vi "Convert CAN Frame.vi"(8 "error in (no error)":errorcluster, 9 "timestamp":timestamp, 10 "CAN frame":T1 {"type" items=["CAN Data", "CAN Remote"]; "identifier" format="%.0x"}, 11 "tdms file":refnum<k34>) -> (0 "error out":errorcluster, 3 "tdms file out":refnum<k34>)   [LabVIEW 2014]
uses:
  <vilib>/RioEmbeddedCAN/RioEmbeddedCAN.llb/CANFrameControl.ctl
  TDMS Timestamp and Data Double.vi
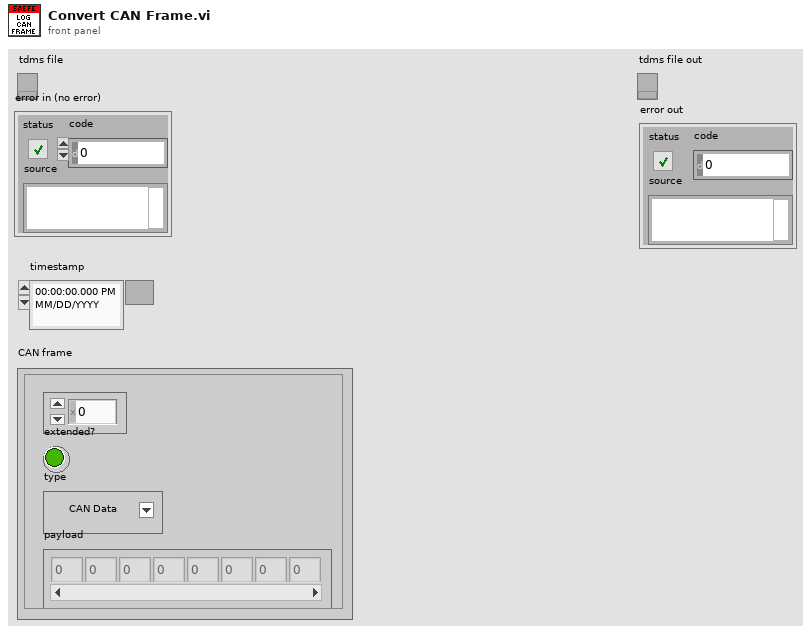
[diagram p1: front panel]
types:
  T1 = typedef "CANFrameControl.ctl" = cluster{"identifier":u32, "extended?":bool, "type":u8, "payload":u8[]}
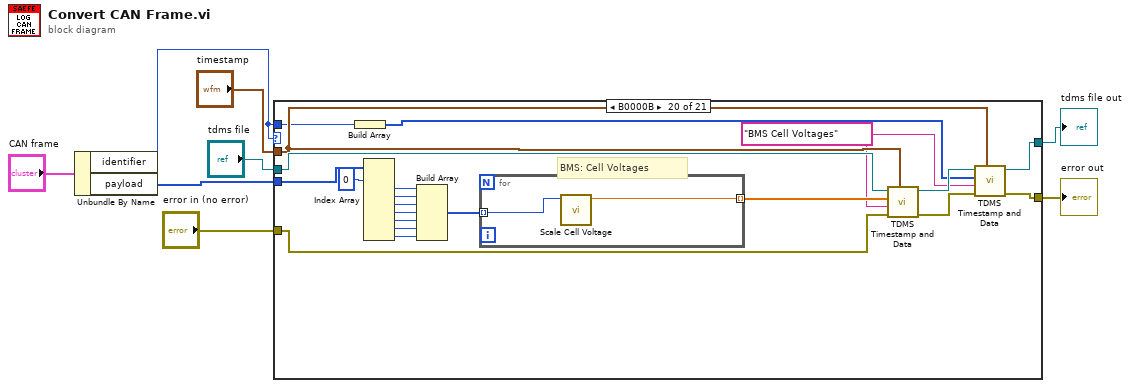
[diagram p0: block diagram]
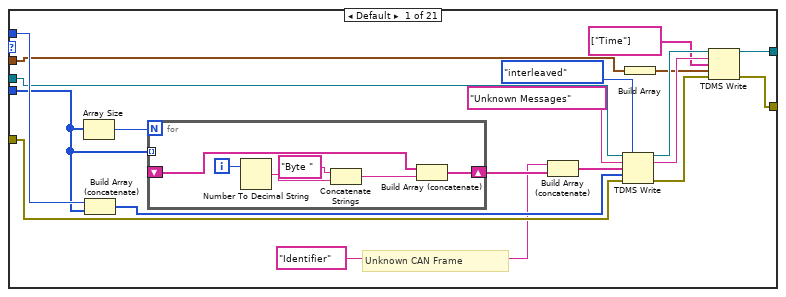
[diagram p2: hidden frame]
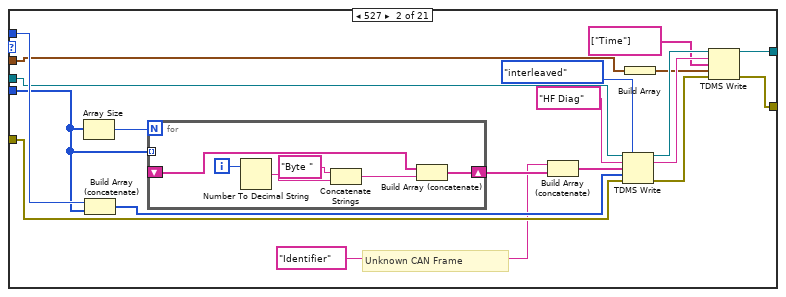
[diagram p3: hidden frame]
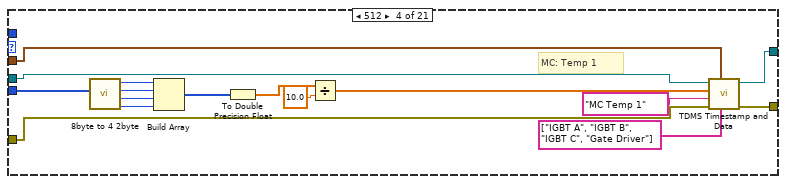
[diagram p5: hidden frame]
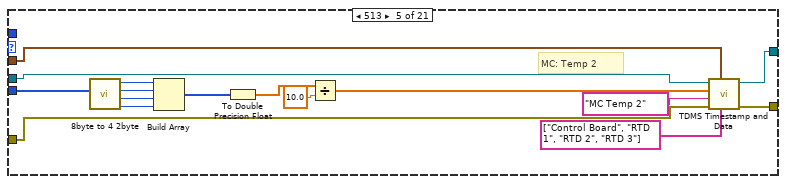
[diagram p6: hidden frame]
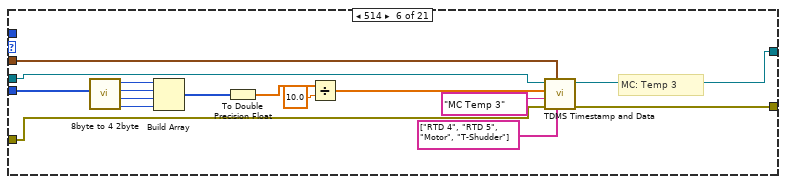
[diagram p7: hidden frame]
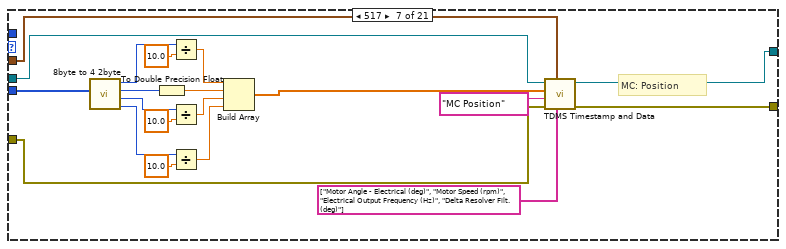
[diagram p8: hidden frame]
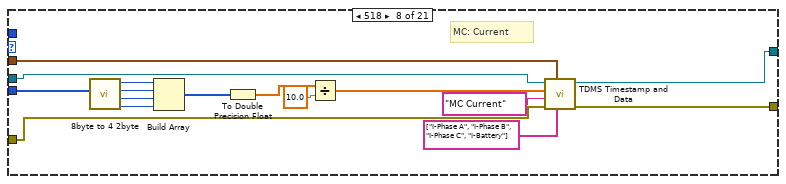
[diagram p9: hidden frame]
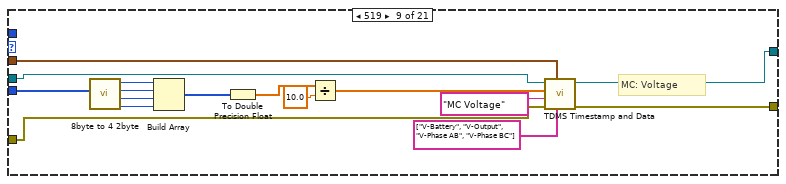
[diagram p10: hidden frame]
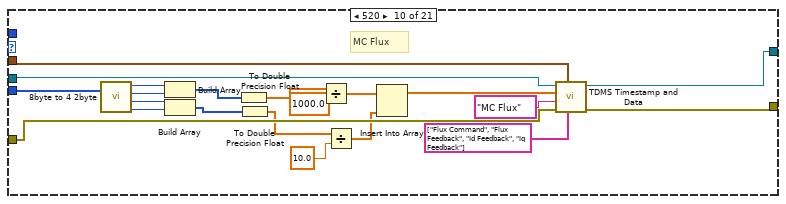
[diagram p11: hidden frame]
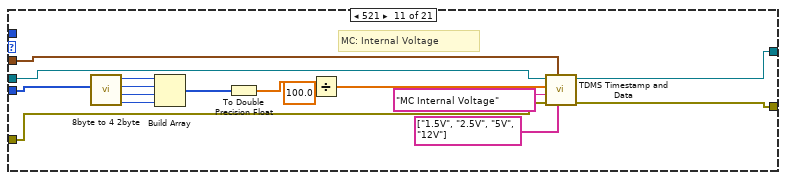
[diagram p12: hidden frame]
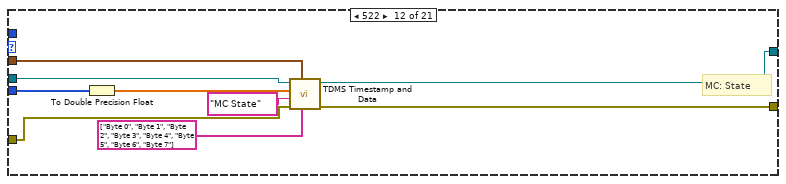
[diagram p13: hidden frame]
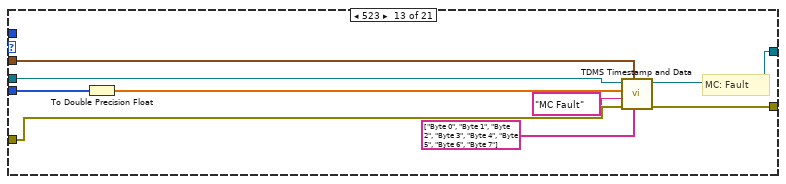
[diagram p14: hidden frame]
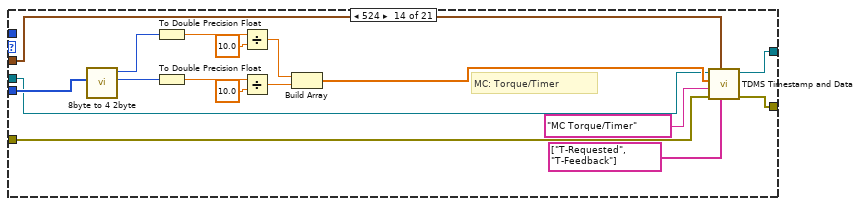
[diagram p15: hidden frame]
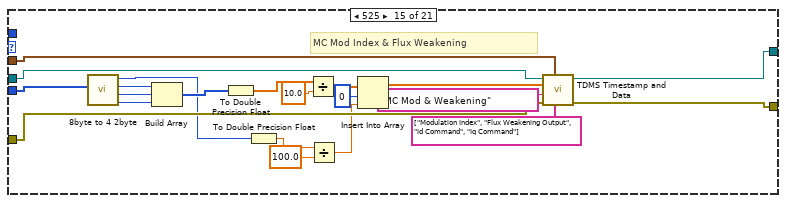
[diagram p16: hidden frame]
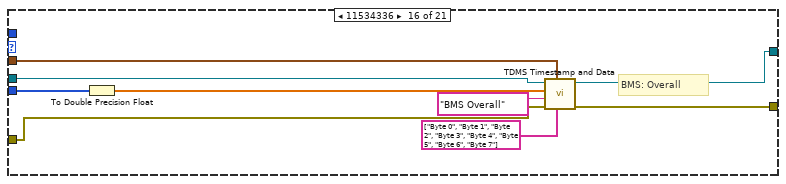
[diagram p17: hidden frame]
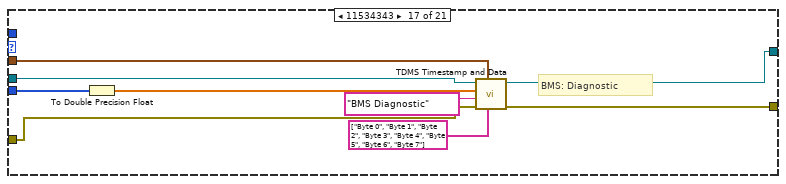
[diagram p18: hidden frame]
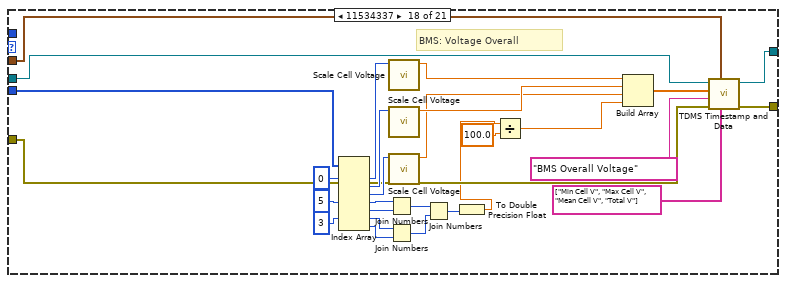
[diagram p19: hidden frame]
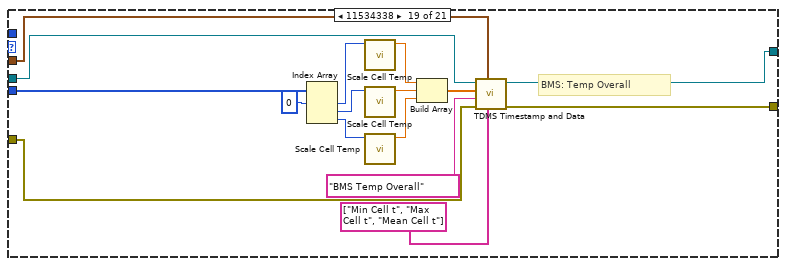
[diagram p20: hidden frame]
diagram:
  n1 = Unbundle By Name("CAN frame") -> ("identifier"=w5:u32, "payload"=w7:u8[])
  n2 = case shown="B0000B" w5 {
    tunnel: w5 -> [w27 w52 _ _ _ _ _ _ _ _ _ _ _ _ _ _ _ _ _ w320 w340]
    tunnel: w7 -> [w9 w34 _ w76 w92 w108 w128 w144 w160 w172 w184 w206 w215 w232 w243 w259 w268 w299 w315 w325 w348]
    tunnel: "timestamp" -> [w14 w39 _ w62 w84 w98 w116 w134 w149 w174 w186 w205 w212 w221 w245 w260 w269 w286 w310 w321 w342]
    tunnel: "tdms file" -> [w26 w51 w60 w68 w83 w99 w115 w136 w152 w173 w185 w204 w213 w222 w244 w262 w271 w288 w309 w327 w350]
    tunnel: [w11 w36 w60 w65 w80 w96 w112 w130 w147 w170 w183 w201 w209 w218 w241 w256 w265 w284 w301 w317 w344] -> w3
    tunnel: "error in (no error)" -> [w25 w50 w59 w61 w82 w97 w114 w135 w151 w171 w187 w203 w211 w220 w242 w261 w270 w287 w308 w326 w349]
    tunnel: [w12 w37 w59 w64 w81 w95 w113 w129 w146 w169 w182 w200 w208 w217 w240 w255 w264 w283 w300 w316 w343] -> w1
    frame Default {
      # "Unknown CAN Frame"
      n3 = Array Size(array=w9) -> (size(s)=w10:i32)
      n4 = Build Array (concatenate)(w27, w9) -> (w24:u32[])
      n5 = for {
        N: w10 -> [_]
        tunnel: w9 -> [_] mode=indexing
        shift-right: [w32] -> w23
        shift-left: _ -> [w28]
        i -> [w31]
        n6 = Number To Decimal String(number=w31) -> (decimal integer string=w30:string)  [unwired: 1 in]
        n7 = Concatenate Strings("Byte " ("string"), w30) -> (w33:string)
        n8 = Build Array (concatenate)(w28, w33) -> (w32:string[])
      }
      n9 = Build Array (concatenate)("Identifier", w23) -> (w21:string[])
      n10 = TDMS Write(0:w26, 1:enum16{"decimated", "interleaved"}."interleaved" ("data layout (0:decimated)"), 5:"Unknown Messages" ("group name in (Untitled)"), 7:w21, 9:w24, 11:w25) -> (4:w18:refnum<k34>, 6:w16:string, 15:w17:errorcluster)  [unwired: 1 out]
      n11 = Build Array(w14) -> (w13:timestamp[])
      n12 = TDMS Write(0:w18, 5:w16, 7:string[] ["Time"] ("channel name(s) in (Untitled)"), 9:w13, 11:w17) -> (4:w11:refnum<k34>, 15:w12:errorcluster)  [unwired: 1 in, 2 out]
    }
    frame 527 {
      # "Unknown CAN Frame"
      n13 = Array Size(array=w34) -> (size(s)=w35:i32)
      n14 = Build Array (concatenate)(w52, w34) -> (w49:u32[])
      n15 = for {
        N: w35 -> [_]
        tunnel: w34 -> [_] mode=indexing
        shift-right: [w57] -> w48
        shift-left: _ -> [w53]
        i -> [w56]
        n16 = Number To Decimal String(number=w56) -> (decimal integer string=w55:string)  [unwired: 1 in]
        n17 = Concatenate Strings("Byte " ("string"), w55) -> (w58:string)
        n18 = Build Array (concatenate)(w53, w58) -> (w57:string[])
      }
      n19 = Build Array (concatenate)("Identifier", w48) -> (w46:string[])
      n20 = TDMS Write(0:w51, 1:enum16{"decimated", "interleaved"}."interleaved" ("data layout (0:decimated)"), 5:"HF Diag" ("group name in (Untitled)"), 7:w46, 9:w49, 11:w50) -> (4:w43:refnum<k34>, 6:w41:string, 15:w42:errorcluster)  [unwired: 1 out]
      n21 = Build Array(w39) -> (w38:timestamp[])
      n22 = TDMS Write(0:w43, 5:w41, 7:string[] ["Time"] ("channel name(s) in (Untitled)"), 9:w38, 11:w42) -> (4:w36:refnum<k34>, 15:w37:errorcluster)  [unwired: 1 in, 2 out]
    }
    frame 0 {
      # "Do nothing for NULL frame"
    }
    frame 512 {
      # "MC: Temp 1"
      n23 = call "8byte to 4 2byte.vi"("payload"=w76) -> ("7,6"=w72:i16, "5,4"=w73:i16, "3,2"=w74:i16, "1,0"=w75:i16)  [unwired: 7 in]
      n24 = Build Array(w75, w74, w73, w72) -> (w69:i16[])
      n25 = To Double Precision Float(number=w69) -> (double precision float=w70:dbl[])
      n26 = Divide(x=w70, y=10.0) -> (x/y=w63:dbl[])
      n27 = call-poly "TDMS Timestamp and Data.vi"("channel name(s) in (Untitled)"=string[] ["IGBT A", "IGBT B", "IGBT C", "Gate Driver"], "timestamp"=w62, "error in (no error)"=w61, "group name in (Untitled)"="MC Temp 1", "Array"=w63, "Refnum in"=w68) -> ("error out"=w64:errorcluster, "Refnum out"=w65:refnum<k34>)  [unwired: 4 in]
    }
    frame 513 {
      # "MC: Temp 2"
      n28 = call "8byte to 4 2byte.vi"("payload"=w92) -> ("7,6"=w88:i16, "5,4"=w89:i16, "3,2"=w90:i16, "1,0"=w91:i16)  [unwired: 7 in]
      n29 = Build Array(w91, w90, w89, w88) -> (w85:i16[])
      n30 = To Double Precision Float(number=w85) -> (double precision float=w86:dbl[])
      n31 = Divide(x=w86, y=10.0) -> (x/y=w79:dbl[])
      n32 = call-poly "TDMS Timestamp and Data.vi"("channel name(s) in (Untitled)"=string[] ["Control Board", "RTD 1", "RTD 2", "RTD 3"], "timestamp"=w84, "error in (no error)"=w82, "group name in (Untitled)"="MC Temp 2", "Array"=w79, "Refnum in"=w83) -> ("error out"=w81:errorcluster, "Refnum out"=w80:refnum<k34>)  [unwired: 4 in]
    }
    frame 514 {
      # "MC: Temp 3"
      n33 = call "8byte to 4 2byte.vi"("payload"=w108) -> ("7,6"=w104:i16, "5,4"=w105:i16, "3,2"=w106:i16, "1,0"=w107:i16)  [unwired: 7 in]
      n34 = Build Array(w107, w106, w105, w104) -> (w101:i16[])
      n35 = To Double Precision Float(number=w101) -> (double precision float=w102:dbl[])
      n36 = Divide(x=w102, y=10.0) -> (x/y=w100:dbl[])
      n37 = call-poly "TDMS Timestamp and Data.vi"("channel name(s) in (Untitled)"=string[] ["RTD 4", "RTD 5", "Motor", "T-Shudder"], "timestamp"=w98, "error in (no error)"=w97, "group name in (Untitled)"="MC Temp 3", "Array"=w100, "Refnum in"=w99) -> ("error out"=w95:errorcluster, "Refnum out"=w96:refnum<k34>)  [unwired: 4 in]
    }
    frame 517 {
      # "MC: Position"
      n38 = call "8byte to 4 2byte.vi"("payload"=w128) -> ("7,6"=w123:i16, "5,4"=w124:i16, "3,2"=w118:i16, "1,0"=w127:i16)  [unwired: 7 in]
      n39 = To Double Precision Float(number=w118) -> (double precision float=w117:dbl)
      n40 = Divide(x=w127, y=10.0) -> (x/y=w122:dbl)
      n41 = Divide(x=w124, y=10.0) -> (x/y=w121:dbl)
      n42 = Divide(x=w123, y=10.0) -> (x/y=w120:dbl)
      n43 = Build Array(w122, w117, w121, w120) -> (w109:dbl[])
      n44 = call-poly "TDMS Timestamp and Data.vi"("channel name(s) in (Untitled)"=string[] ["Motor Angle - Electrical (deg)", "Motor Speed (rpm)", "Electrical Output Frequency (Hz)", "Delta Resolver Filt. (deg)"], "timestamp"=w116, "error in (no error)"=w114, "group name in (Untitled)"="MC Position", "Array"=w109, "Refnum in"=w115) -> ("error out"=w113:errorcluster, "Refnum out"=w112:refnum<k34>)  [unwired: 4 in]
    }
    frame 518 {
      # "MC: Current"
      n45 = call "8byte to 4 2byte.vi"("payload"=w144) -> ("7,6"=w140:i16, "5,4"=w141:i16, "3,2"=w142:i16, "1,0"=w143:i16)  [unwired: 7 in]
      n46 = Build Array(w143, w142, w141, w140) -> (w137:i16[])
      n47 = To Double Precision Float(number=w137) -> (double precision float=w138:dbl[])
      n48 = Divide(x=w138, y=10.0) -> (x/y=w133:dbl[])
      n49 = call-poly "TDMS Timestamp and Data.vi"("channel name(s) in (Untitled)"=string[] ["I-Phase A", "I-Phase B", "I-Phase C", "I-Battery"], "timestamp"=w134, "error in (no error)"=w135, "group name in (Untitled)"="MC Current", "Array"=w133, "Refnum in"=w136) -> ("error out"=w129:errorcluster, "Refnum out"=w130:refnum<k34>)  [unwired: 4 in]
    }
    frame 519 {
      # "MC: Voltage"
      n50 = call "8byte to 4 2byte.vi"("payload"=w160) -> ("7,6"=w156:i16, "5,4"=w157:i16, "3,2"=w158:i16, "1,0"=w159:i16)  [unwired: 7 in]
      n51 = Build Array(w159, w158, w157, w156) -> (w153:i16[])
      n52 = To Double Precision Float(number=w153) -> (double precision float=w154:dbl[])
      n53 = Divide(x=w154, y=10.0) -> (x/y=w150:dbl[])
      n54 = call-poly "TDMS Timestamp and Data.vi"("channel name(s) in (Untitled)"=string[] ["V-Battery", "V-Output", "V-Phase AB", "V-Phase BC"], "timestamp"=w149, "error in (no error)"=w151, "group name in (Untitled)"="MC Voltage", "Array"=w150, "Refnum in"=w152) -> ("error out"=w146:errorcluster, "Refnum out"=w147:refnum<k34>)  [unwired: 4 in]
    }
    frame 520 {
      # "MC Flux"
      n55 = call "8byte to 4 2byte.vi"("payload"=w172) -> ("7,6"=w167:i16, "5,4"=w168:i16, "3,2"=w180:i16, "1,0"=w181:i16)  [unwired: 7 in]
      n56 = Build Array(w181, w180) -> (w177:i16[])
      n57 = Build Array(w168, w167) -> (w166:i16[])
      n58 = To Double Precision Float(number=w177) -> (double precision float=w178:dbl[])
      n59 = To Double Precision Float(number=w166) -> (double precision float=w165:dbl[])
      n60 = Divide(x=w178, y=1000.0) -> (x/y=w163:dbl[])
      n61 = Divide(x=w165, y=10.0 ("7,6")) -> (x/y=w162:dbl[])
      n62 = Insert Into Array(array=w163, new element=w162) -> (w161:dbl[])  [unwired: 1 in]
      n63 = call-poly "TDMS Timestamp and Data.vi"("channel name(s) in (Untitled)"=string[] ["Flux Command", "Flux Feedback", "Id Feedback", "Iq Feedback"], "timestamp"=w174, "error in (no error)"=w171, "group name in (Untitled)"="MC Flux", "Array"=w161, "Refnum in"=w173) -> ("error out"=w169:errorcluster, "Refnum out"=w170:refnum<k34>)  [unwired: 4 in]
    }
    frame 521 {
      # "MC: Internal Voltage"
      n64 = call "8byte to 4 2byte.vi"("payload"=w184) -> ("7,6"=w194:i16, "5,4"=w195:i16, "3,2"=w196:i16, "1,0"=w197:i16)  [unwired: 7 in]
      n65 = Build Array(w197, w196, w195, w194) -> (w191:i16[])
      n66 = To Double Precision Float(number=w191) -> (double precision float=w192:dbl[])
      n67 = Divide(x=w192, y=100.0) -> (x/y=w190:dbl[])
      n68 = call-poly "TDMS Timestamp and Data.vi"("channel name(s) in (Untitled)"=string[] ["1.5V", "2.5V", "5V", "12V"], "timestamp"=w186, "error in (no error)"=w187, "group name in (Untitled)"="MC Internal Voltage", "Array"=w190, "Refnum in"=w185) -> ("error out"=w182:errorcluster, "Refnum out"=w183:refnum<k34>)  [unwired: 4 in]
    }
    frame 522 {
      # "MC: State"
      n69 = To Double Precision Float(number=w206) -> (double precision float=w202:dbl[])
      n70 = call-poly "TDMS Timestamp and Data.vi"("channel name(s) in (Untitled)"=string[] ["Byte 0", "Byte 1", "Byte 2", "Byte 3", "Byte 4", "Byte 5", "Byte 6", "Byte 7"], "timestamp"=w205, "error in (no error)"=w203, "group name in (Untitled)"="MC State", "Array"=w202, "Refnum in"=w204) -> ("error out"=w200:errorcluster, "Refnum out"=w201:refnum<k34>)  [unwired: 4 in]
    }
    frame 523 {
      # "MC: Fault"
      n71 = To Double Precision Float(number=w215) -> (double precision float=w214:dbl[])
      n72 = call-poly "TDMS Timestamp and Data.vi"("channel name(s) in (Untitled)"=string[] ["Byte 0", "Byte 1", "Byte 2", "Byte 3", "Byte 4", "Byte 5", "Byte 6", "Byte 7"], "timestamp"=w212, "error in (no error)"=w211, "group name in (Untitled)"="MC Fault", "Array"=w214, "Refnum in"=w213) -> ("error out"=w208:errorcluster, "Refnum out"=w209:refnum<k34>)  [unwired: 4 in]
    }
    frame 524 {
      # "MC: Torque/Timer"
      n73 = call "8byte to 4 2byte.vi"("payload"=w232) -> ("3,2"=w228:i16, "1,0"=w231:i16)  [unwired: 7 in, 2 out]
      n74 = To Double Precision Float(number=w231) -> (double precision float=w230:dbl)
      n75 = To Double Precision Float(number=w228) -> (double precision float=w227:dbl)
      n76 = Divide(x=w230, y=10.0) -> (x/y=w225:dbl)
      n77 = Divide(x=w227, y=10.0) -> (x/y=w224:dbl)
      n78 = Build Array(w225, w224) -> (w223:dbl[])
      n79 = call-poly "TDMS Timestamp and Data.vi"("channel name(s) in (Untitled)"=string[] ["T-Requested", "T-Feedback"], "timestamp"=w221, "error in (no error)"=w220, "group name in (Untitled)"="MC Torque/Timer", "Array"=w223, "Refnum in"=w222) -> ("error out"=w217:errorcluster, "Refnum out"=w218:refnum<k34>)  [unwired: 4 in]
    }
    frame 525 {
      # "MC Mod Index & Flux Weakening"
      n80 = call "8byte to 4 2byte.vi"("payload"=w243) -> ("7,6"=w248:i16, "5,4"=w247:i16, "3,2"=w246:i16, "1,0"=w237:i16)  [unwired: 7 in]
      n81 = Build Array(w246, w247, w248) -> (w251:i16[])
      n82 = To Double Precision Float(number=w251) -> (double precision float=w250:dbl[])
      n83 = To Double Precision Float(number=w237) -> (double precision float=w235:dbl)
      n84 = Divide(x=w250, y=10.0) -> (x/y=w239:dbl[])
      n85 = Divide(x=w235, y=100.0) -> (x/y=w234:dbl)
      n86 = Insert Into Array(array=w239, index=0, new element=w234) -> (w236:dbl[])
      n87 = call-poly "TDMS Timestamp and Data.vi"("channel name(s) in (Untitled)"=string[] ["Modulation Index", "Flux Weakening Output", "Id Command", "Iq Command"], "timestamp"=w245, "error in (no error)"=w242, "group name in (Untitled)"="MC Mod & Weakening", "Array"=w236, "Refnum in"=w244) -> ("error out"=w240:errorcluster, "Refnum out"=w241:refnum<k34>)  [unwired: 4 in]
    }
    frame 11534336 {
      # "BMS: Overall"
      n88 = To Double Precision Float(number=w259) -> (double precision float=w258:dbl[])
      n89 = call-poly "TDMS Timestamp and Data.vi"("channel name(s) in (Untitled)"=string[] ["Byte 0", "Byte 1", "Byte 2", "Byte 3", "Byte 4", "Byte 5", "Byte 6", "Byte 7"], "timestamp"=w260, "error in (no error)"=w261, "group name in (Untitled)"="BMS Overall", "Array"=w258, "Refnum in"=w262) -> ("error out"=w255:errorcluster, "Refnum out"=w256:refnum<k34>)  [unwired: 4 in]
    }
    frame 11534343 {
      # "BMS: Diagnostic"
      n90 = To Double Precision Float(number=w268) -> (double precision float=w267:dbl[])
      n91 = call-poly "TDMS Timestamp and Data.vi"("channel name(s) in (Untitled)"=string[] ["Byte 0", "Byte 1", "Byte 2", "Byte 3", "Byte 4", "Byte 5", "Byte 6", "Byte 7"], "timestamp"=w269, "error in (no error)"=w270, "group name in (Untitled)"="BMS Diagnostic", "Array"=w267, "Refnum in"=w271) -> ("error out"=w264:errorcluster, "Refnum out"=w265:refnum<k34>)  [unwired: 4 in]
    }
    frame 11534337 {
      # "BMS: Voltage Overall"
      n92 = Index Array(array=w299, index #1=0 ("index"), index #4=5 ("index"), index #6=3 ("index")) -> (element #1=w297:u8, element #2=w296:u8, element #3=w295:u8, element #4=w280:u8, element #5=w279:u8, element #6=w275:u8, element #7=w274:u8)  [unwired: 4 in]
      n93 = Join Numbers(hi=w280, lo=w279) -> ((hi.lo)=w276:u16)
      n94 = Join Numbers(hi=w275, lo=w274) -> ((hi.lo)=w277:u16)
      n95 = call "Scale Cell Voltage.vi"("Numeric in"=w297) -> ("Numeric out"=w293:dbl)  [unwired: 10 in]
      n96 = call "Scale Cell Voltage.vi"("Numeric in"=w296) -> ("Numeric out"=w292:dbl)  [unwired: 10 in]
      n97 = call "Scale Cell Voltage.vi"("Numeric in"=w295) -> ("Numeric out"=w291:dbl)  [unwired: 10 in]
      n98 = Join Numbers(hi=w276, lo=w277) -> ((hi.lo)=w273:u32)
      n99 = To Double Precision Float(number=w273) -> (double precision float=w272:dbl)
      n100 = Divide(x=w272, y=100.0) -> (x/y=w290:dbl)
      n101 = Build Array(w293, w292, w291, w290) -> (w289:dbl[])
      n102 = call-poly "TDMS Timestamp and Data.vi"("channel name(s) in (Untitled)"=string[] ["Min Cell V", "Max Cell V", "Mean Cell V", "Total V"], "timestamp"=w286, "error in (no error)"=w287, "group name in (Untitled)"="BMS Overall Voltage", "Array"=w289, "Refnum in"=w288) -> ("error out"=w283:errorcluster, "Refnum out"=w284:refnum<k34>)  [unwired: 4 in]
    }
    frame 11534338 {
      # "BMS: Temp Overall"
      n103 = Index Array(array=w315, index #1=0 ("index")) -> (element #1=w313:u8, element #2=w312:u8, element #3=w311:u8)  [unwired: 2 in]
      n104 = call "Scale Cell Temp.vi"("Numeric in"=w313) -> ("Numeric out"=w307:dbl)  [unwired: 10 in]
      n105 = call "Scale Cell Temp.vi"("Numeric in"=w312) -> ("Numeric out"=w306:dbl)  [unwired: 10 in]
      n106 = call "Scale Cell Temp.vi"("Numeric in"=w311) -> ("Numeric out"=w305:dbl)  [unwired: 10 in]
      n107 = Build Array(w307, w306, w305) -> (w304:dbl[])
      n108 = call-poly "TDMS Timestamp and Data.vi"("channel name(s) in (Untitled)"=string[] ["Min Cell t", "Max Cell t", "Mean Cell t"], "timestamp"=w310, "error in (no error)"=w308, "group name in (Untitled)"="BMS Temp Overall", "Array"=w304, "Refnum in"=w309) -> ("error out"=w300:errorcluster, "Refnum out"=w301:refnum<k34>)  [unwired: 4 in]
    }
    frame 11534347 {
      w318 = "BMS Cell Voltages" ("group name in (Untitled)")
      # "BMS: Cell Voltages"
      n109 = Build Array(w320) -> (w319:u32[])
      n110 = Index Array(array=w325, index #1=0 ("index")) -> (element #2=w335:u8, element #3=w334:u8, element #4=w333:u8, element #5=w332:u8, element #6=w331:u8, element #7=w330:u8, element #8=w329:u8)  [unwired: 7 in, 1 out]
      n111 = Build Array(w335, w334, w333, w332, w331, w330, w329) -> (w328:u8[])
      n112 = for {
        tunnel: w328 -> [w338] mode=indexing
        tunnel: [w337] -> w324 mode=indexing
        n113 = call "Scale Cell Voltage.vi"("Numeric in"=w338) -> ("Numeric out"=w337:dbl)  [unwired: 10 in]
      }
      n114 = call-poly "TDMS Timestamp and Data.vi"("timestamp"=w321, "error in (no error)"=w326, "group name in (Untitled)"=w318, "Array"=w324, "Refnum in"=w327) -> ("error out"=w322:errorcluster, "Refnum out"=w323:refnum<k34>)  [unwired: 5 in]
      n115 = call-poly "TDMS Timestamp and Data.vi"("timestamp"=w321, "error in (no error)"=w322, "group name in (Untitled)"=w318, "Array"=w319, "Refnum in"=w323) -> ("error out"=w316:errorcluster, "Refnum out"=w317:refnum<k34>)  [unwired: 5 in]
    }
    frame 11534348 {
      w341 = "BMS Cell Temps" ("group name in (Untitled)")
      # "BMS: Cell Temps"
      n116 = Build Array(w340) -> (w339:u32[])
      n117 = Index Array(array=w348, index #1=0 ("index")) -> (element #2=w358:u8, element #3=w357:u8, element #4=w356:u8, element #5=w355:u8, element #6=w354:u8, element #7=w353:u8, element #8=w352:u8)  [unwired: 7 in, 1 out]
      n118 = Build Array(w358, w357, w356, w355, w354, w353, w352) -> (w351:u8[])
      n119 = for {
        tunnel: w351 -> [w360] mode=indexing
        tunnel: [w361] -> w347 mode=indexing
        n120 = call "Scale Cell Temp.vi"("Numeric in"=w360) -> ("Numeric out"=w361:dbl)  [unwired: 10 in]
      }
      n121 = call-poly "TDMS Timestamp and Data.vi"("timestamp"=w342, "error in (no error)"=w349, "group name in (Untitled)"=w341, "Array"=w347, "Refnum in"=w350) -> ("error out"=w345:errorcluster, "Refnum out"=w346:refnum<k34>)  [unwired: 5 in]
      n122 = call-poly "TDMS Timestamp and Data.vi"("timestamp"=w342, "error in (no error)"=w345, "group name in (Untitled)"=w341, "Array"=w339, "Refnum in"=w346) -> ("error out"=w343:errorcluster, "Refnum out"=w344:refnum<k34>)  [unwired: 5 in]
    }
  }
  "tdms file out" <- w3
  "error out" <- w1
